vi "String_ShowScrollBar.vi"(8 "error in (no error)":errorcluster, 9 "hide control if empty text":bool, 10 "new text":string, 11 "dialog string refnum":refnum<vi>) -> (0 "error out":errorcluster)   [LabVIEW 2017]
doc: "This utility will show or hide the vertical scrollbar based on the size of the text. It assumes the reference is to a dialog string control, as it doesn't account for different fonts or control border pixels."
panel:
  in  "dummy":string
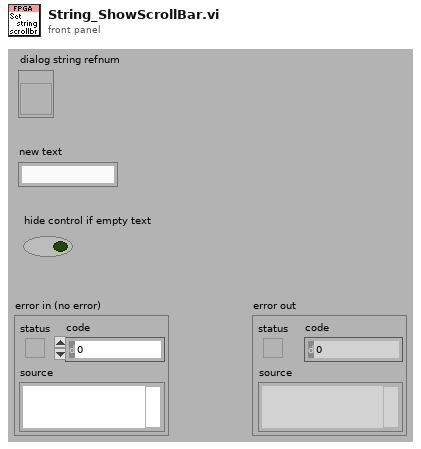
[diagram p1: front panel]
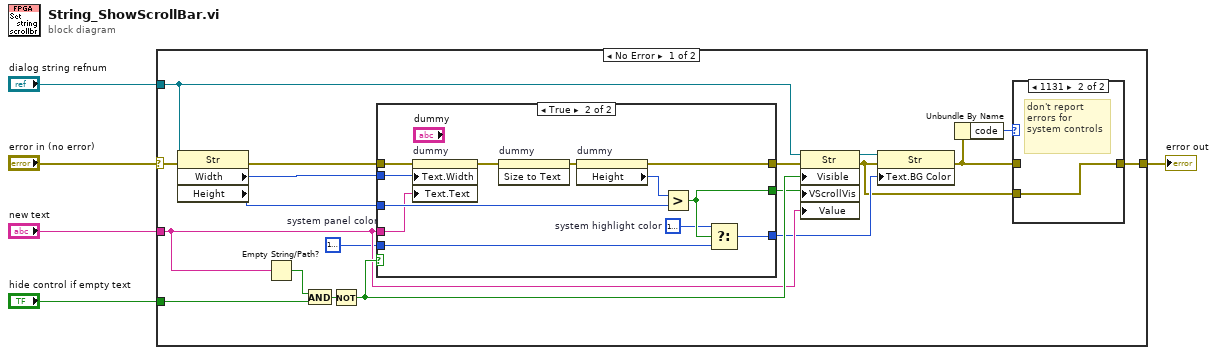
[diagram p0: block diagram]
diagram:
  n1 = case shown="No Error" "error in (no error)" {
    selector: "error in (no error)" -> [w14 w41]
    tunnel: "hide control if empty text" -> [w19 _]
    tunnel: [w8 w41] -> w4
    tunnel: "dialog string refnum" -> [w15 _]
    tunnel: "new text" -> [w13 _]
    frame No Error {
      w6 = u32 16777238  # system panel color
      n2 = property class="Str"(reference=w15, error in=w14) -> (error out=w22:errorcluster, "Width"=w24:u32, "Height"=w23:u32)  [unwired: 1 out]
      n3 = Empty String/Path?(string/path=w13) -> (empty?=w18:bool)
      n4 = And(x=w18, y=w19) -> (x .and. y?=w20:bool)
      n5 = Not(x=w20) -> (.not. x?=w17:bool)
      n6 = case shown="True" w17 {
        tunnel: w24 -> [_ w40]
        tunnel: w23 -> [_ w39]
        tunnel: w22 -> [w28 w35]
        tunnel: [w28 w34] -> w21
        tunnel: w13 -> [_ w33]
        tunnel: [_ w32] -> w16
        tunnel: [w27 w30] -> w12
        tunnel: w6 -> [w27 w29]
        frame False {
        }
        frame True {
          w31 = u32 16777224  # system highlight color
          n7 = property on="dummy" class="Str"(error in=w35, "Text.Width"=w40, "Text.Text"=w33) -> (error out=w38:errorcluster)  [unwired: 1 in, 1 out]
          n8 = invoke on="dummy" class="Str" method="Size to Text"(error in=w38) -> (error out=w37:errorcluster)  [unwired: 2 in, 2 out]
          n9 = property on="dummy" class="Str"(error in=w37) -> (error out=w34:errorcluster, "Height"=w36:u32)  [unwired: 1 in, 1 out]
          n10 = Greater?(x=w36, y=w39) -> (0:w32:bool)
          n11 = Select(t=w31, s=w32, f=w29) -> (s? t:f=w30:u32)
        }
      }
      n12 = property class="Str"(reference=w15, error in=w21, "Visible"=w17, "VScrollVis"=w16, "Value"=w13) -> (reference out=w11:refnum<vi>, error out=w9:errorcluster)
      n13 = property class="Str"(reference=w11, error in=w9, "Text.BG Color"=w12) -> (error out=w7:errorcluster)  [unwired: 1 out]
      n14 = Unbundle By Name(w7) -> ("code"=w10:i32)
      n15 = case shown="1131" w10 {
        tunnel: [w25 w26] -> w8
        tunnel: w9 -> [_ w26]
        tunnel: w7 -> [w25 _]
        frame Default {
        }
        frame 1131 {
          # "don't report errors for system controls"
        }
      }
    }
    frame Error {
    }
  }
  "error out" <- w4
